vi "GetValue.vi"(8 "error in":errorcluster, 11 "Boolean in":refnum<class "Boolean.lvclass">) -> (0 "error out":errorcluster, 2 "Value":bool, 3 "Boolean out":refnum<class "Boolean.lvclass">)   [LabVIEW 2021, in "ProligentXMLGenerator.lvlib" / "Boolean.lvclass"]
uses:
  Boolean.lvclass
  Boolean.lvclass/Boolean.ctl
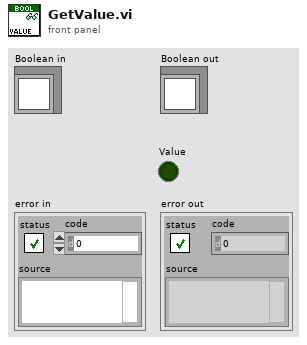
[diagram p1: front panel]
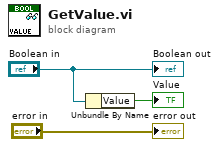
[diagram p0: block diagram]
diagram:
  n1 = Unbundle By Name("Boolean in") -> ("Value"=→"Value":bool)
  "error out" <- "error in"
  "Boolean out" <- "Boolean in"
